vi "SetSelectRowColor(MultList).vi"(9 "OthersRow":u32(colorbox)=16448250, 10 "SelectRow":u32(colorbox)=12369084, 11 "MultList输入":refnum<vi>) -> ()   [LabVIEW 2018]
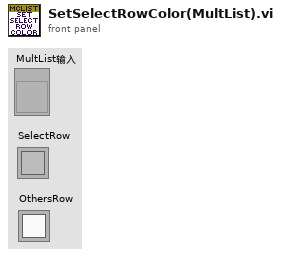
[diagram p1: front panel]
types:
  T1 = typedef "LVRowAndColumnTypeDef.ctl" = cluster{"Row":i32, "Column":i32}
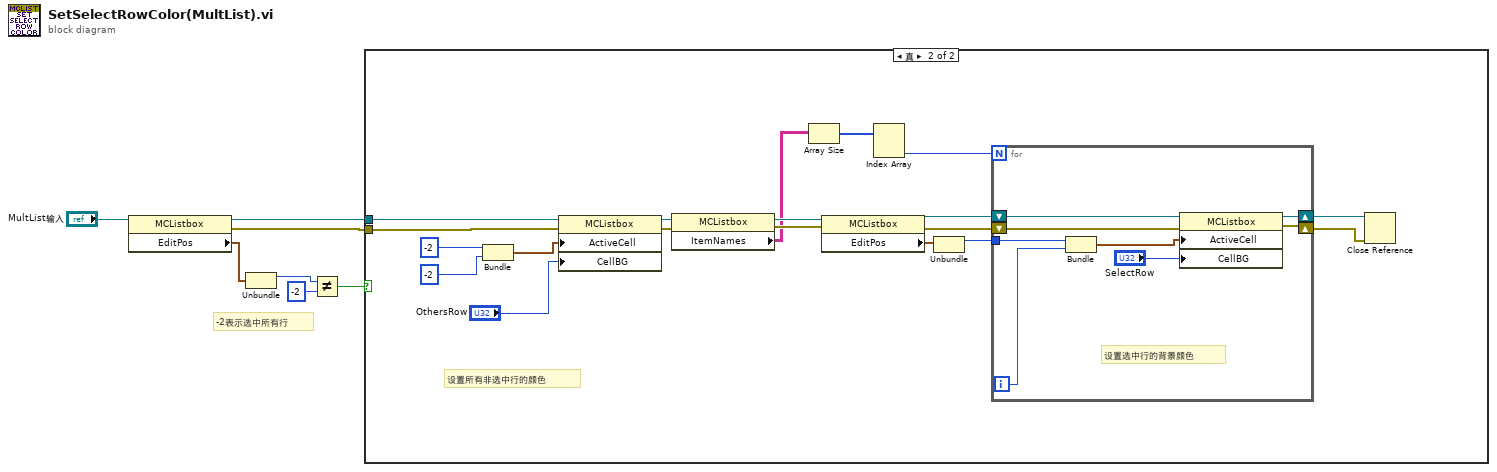
[diagram p0: block diagram]
diagram:
  # "-2表示选中所有行"
  n1 = property class="MCListbox"(reference="MultList输入") -> (reference out=w6:refnum<vi>, error out=w3:errorcluster, "EditPos"=w2:T1)  [unwired: 1 in]
  n2 = Unbundle(w2) -> ("Row"=w1:i32)  [unwired: 1 out]
  n3 = Not Equal?(x=w1, y=-2) -> (x != y?=w4:bool)
  n4 = case shown="真" w4 {
    tunnel: w6 -> [_ w18]
    tunnel: w3 -> [_ w17]
    frame False {
    }
    frame True {
      # "设置所有非选中行的颜色"
      n5 = Bundle(-2, -2) -> (w12:cluster{i32, i32})  [unwired: 1 in]
      n6 = property class="MCListbox"(reference=w18, error in=w17, "ActiveCell"=w12, "CellBG"="OthersRow") -> (reference out=w16:refnum<vi>, error out=w15:errorcluster)
      n7 = property class="MCListbox"(reference=w16, error in=w15) -> (reference out=w14:refnum<vi>, error out=w13:errorcluster, "ItemNames"=w11:string[][])
      n8 = Array Size(array=w11) -> (size(s)=w10:i32[])
      n9 = property class="MCListbox"(reference=w14, error in=w13) -> (reference out=w26:refnum<vi>, error out=w25:errorcluster, "EditPos"=w8:T1)
      n10 = Index Array(array=w10) -> (element #2=w9:i32)  [unwired: 2 in, 1 out]
      n11 = Unbundle(w8) -> ("Row"=w24:i32)  [unwired: 1 out]
      n12 = for {
        N: w9 -> [_]
        tunnel: w24 -> [w32]
        shift-right: [w31] -> w23
        shift-left: w26 -> [w34]
        shift-right: [w30] -> w22
        shift-left: w25 -> [w33]
        i -> [w29]
        # "设置选中行的背景颜色"
        n13 = Bundle("Row"=w32, w29) -> (w27:cluster{"Row":i32, i32})  [unwired: 1 in]
        n14 = property class="MCListbox"(reference=w34, error in=w33, "ActiveCell"=w27, "CellBG"="SelectRow") -> (reference out=w31:refnum<vi>, error out=w30:errorcluster)
      }
      n15 = Close Reference(reference=w23, error in (no error)=w22) -> ()  [unwired: 1 out]
    }
  }
